vi "count_Save.vi"(8 "error in (no error)":errorcluster caption="错误输入（无错误）", 9 "R_coutout":string, 10 "R_tota":string, 11 "configuration file path":path caption="配置文件的路径") -> (0 "error out":errorcluster caption="错误输出")   [LabVIEW 2018]
uses:
  <vilib>/Utility/config.llb/Write Key (String).vi
  <vilib>/Utility/config.llb/NI_LVConfig.lvlib
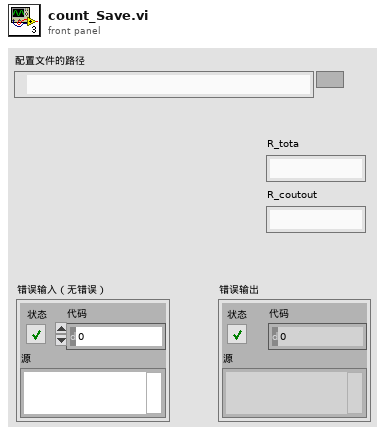
[diagram p1: front panel]
types:
  T1 = typedef "NI_LVConfig.lvlib/Config Data RefNum.ctl" = refnum<k1>
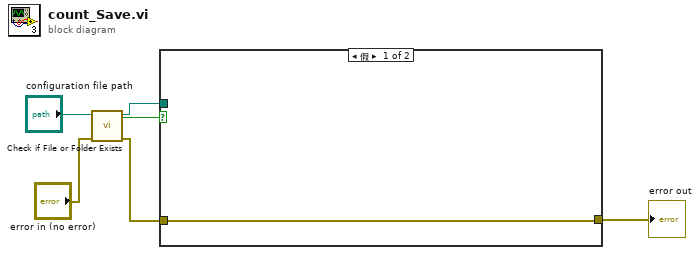
[diagram p0: block diagram]
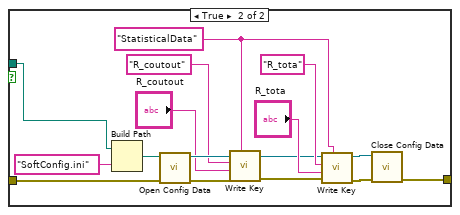
[diagram p2: hidden frame]
diagram:
  n1 = call <vilib>:"Check if File or Folder Exists.vi"("error in (no error)"="error in (no error)", "path"="configuration file path") -> ("error out"=w2:errorcluster, "file or folder exists?"=w5:bool, "dup path"=w4:path)  [unwired: 7 in]
  n2 = case shown="假" w5 {
    tunnel: w4 -> [_ w21]
    tunnel: w2 -> [w7 w10]
    tunnel: [w7 w8] -> w1
    frame False {
    }
    frame True {
      w17 = "StatisticalData" ("section")
      n3 = Build Path(base path=w21, name or relative path="SoftConfig.ini" ("名称或相对路径")) -> (appended path=w23:path)
      n4 = call <vilib>:"Open Config Data.vi"("error in (no error)"=w10, "configuration file path"=w23) -> ("error out"=w9:errorcluster, "refnum"=w20:T1)  [unwired: 7 in, 1 out]
      n5 = call-poly <vilib>:"Write Key.vi"("section"=w17, "error in (no error)"=w9, "value"="R_coutout", "key"="R_coutout", "refnum"=w20) -> ("error out"=w13:errorcluster, "refnum out"=w14:T1)  [unwired: 4 in, 1 out]
      n6 = call-poly <vilib>:"Write Key.vi"("section"=w17, "error in (no error)"=w13, "value"="R_tota", "key"="R_tota", "refnum"=w14) -> ("error out"=w11:errorcluster, "refnum out"=w12:T1)  [unwired: 4 in, 1 out]
      n7 = call <vilib>:"Close Config Data.vi"("error in (no error)"=w11, "refnum"=w12) -> ("error out"=w8:errorcluster)  [unwired: 8 in, 1 out]
    }
  }
  "error out" <- w1
